vi "FPGA_Close.vi"(2 "error in (no error)":errorcluster) -> (0 "error out":errorcluster)   [LabVIEW 2009, in "FPGA.lvlib"]
doc: "Closes the FPGA reference and stops the FPGA code on the target. Needs to be called in the end of the program."
uses:
  FPGA.lvlib
  <vilib>/rvi/interface/nirviCloseFPGA/nirviCloseFPGA.xnode
  FPGA Bitfiles/scmproject.lvproj_FPGA Target_RobotFPGA.vi.lvbitx
  RobotFPGA.vi
  <vilib>/FPGAPlugInAG/cRIO-9074/nirviIntfClose_cRIO-9074.vi
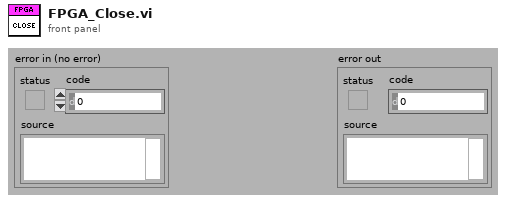
[diagram p1: front panel]
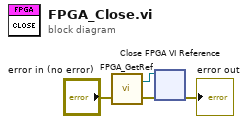
[diagram p0: block diagram]
diagram:
  n1 = call "FPGA_GetRef.vi"("error in (no error)"="error in (no error)") -> ("error out"=w2:errorcluster, "FPGA_Ref"=w3:refnum<k20>)  [unwired: 1 in]
  n2 = xnode "Close FPGA VI Reference"("FPGA VI Reference In"=w3, "error in"=w2) -> ("error out"=→"error out":errorcluster)
